vi "Write to Buffer.vi"(7 "clear buffer (False)":bool, 8 "error in (no error)":errorcluster, 9 "timeout (1000 ms)":i32=1000, 10 "waveforms":waveform(dbl)[](array[waveform]), 11 "buffer":refnum<data-value>) -> (0 "error out":errorcluster, 3 "buffer out":refnum<data-value>)   [LabVIEW 2017, in "Waveforms (N Ch).lvclass"]
doc: "Appends waveforms to existing data in a buffer of continuous waveforms. Use this VI to include additional waveforms in the referenced buffer. <B> waveforms</B> must have identical dt and length, and all waveforms must have the same timestamp. If input waveforms are not continuous with waveforms already in the buffer, the <B> buffer</B> will be cleared and replaced with the <B>waveforms</B>."
uses:
  <vilib>/addons/_NISVFA/_Shared subVIs/Data Objects/Waveforms (DBL)/Waveforms (N Ch).lvclass
  C:/Program Files (x86)/National Instruments/LabVIEW 2017/vi.lib/addons/_NISVFA/_Shared subVIs/Data Objects/Data/Data.lvclass
  <vilib>/addons/_NISVFA/_Shared subVIs/Data Objects/Data/Data.lvclass/Data.ctl
  <vilib>/addons/_NISVFA/_Shared subVIs/Data Objects/Waveforms (DBL)/Waveforms (N Ch).lvclass/Waveforms (N Ch).ctl
  <vilib>/addons/_NISVFA/_Shared subVIs/Data Objects/Waveforms (DBL)/Read Mode for Deleting Stale Data.vi
  <vilib>/addons/_NISVFA/_Shared subVIs/Data Objects/Data/Read Channel Length.vi
  <vilib>/addons/_NISVFA/_Shared subVIs/Data Objects/Waveforms (DBL)/Read Maximum Channel Duration.vi
  <vilib>/addons/_NISVFA/_Shared subVIs/Data Objects/Data/Read Maximum Channel Length.vi
  <vilib>/addons/_NISVFA/_Shared subVIs/Data Objects/Data/Read Channel Count.vi
  <vilib>/addons/_NISVFA/_Shared subVIs/Data Objects/subVIs/Get Oldest of ReaderTimestamps.vi
  <vilib>/addons/_NISVFA/_Shared subVIs/Common/SV Get Data Subset.vi
  <vilib>/addons/_NISVFA/_Shared subVIs/Common/svc_Get Waveform Subset (Index).vi
  <vilib>/addons/_NISVFA/_Shared subVIs/Common/sv_Convert Timestamp to Relative Index.vi
  <vilib>/addons/_NISVFA/_Shared subVIs/Common/sv_Get NI Property Name String.vi
  <vilib>/addons/_NISVFA/_Shared subVIs/Common/svc_Check for Waveform Parameter Continuity (no state).vi
  <vilib>/addons/_NISVFA/_Shared subVIs/Data Objects/subVIs/Get Channel Count.vi
  <vilib>/addons/_NISVFA/_Shared subVIs/Common/svc_Get Array Subset (Index).vi
  <vilib>/addons/_NISVFA/_Shared subVIs/Common/svc_Get SV Channel Info.vi
  <vilib>/addons/_NISVFA/_Shared subVIs/Common/svc_Coerce Index and Length.vi
  <vilib>/addons/_NISVFA/_Shared subVIs/Common/svc_Engineering Units to Unit Label.vi
  <vilib>/addons/_NISVFA/_Shared subVIs/Common/svc_Unit Label to Engineering Units.vi
  <vilib>/addons/_NISVFA/_Shared subVIs/Data Objects/subVIs/Get Maximum Data Length.vi
  <vilib>/addons/_NISVFA/_Shared subVIs/Data Objects/subVIs/Get Maximum Data Duration.vi
  <vilib>/ErrorRing/Error Ring.xnode
  <vilib>/addons/_NISVFA/_Shared subVIs/Data Objects/Data/Data.lvclass
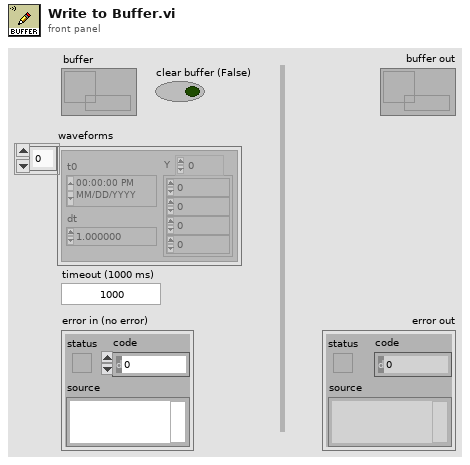
[diagram p1: front panel]
types:
  T1 = typedef "svc_Delete Data Options (enum).ctl" = enum16{"Write", "Read", "Release"}
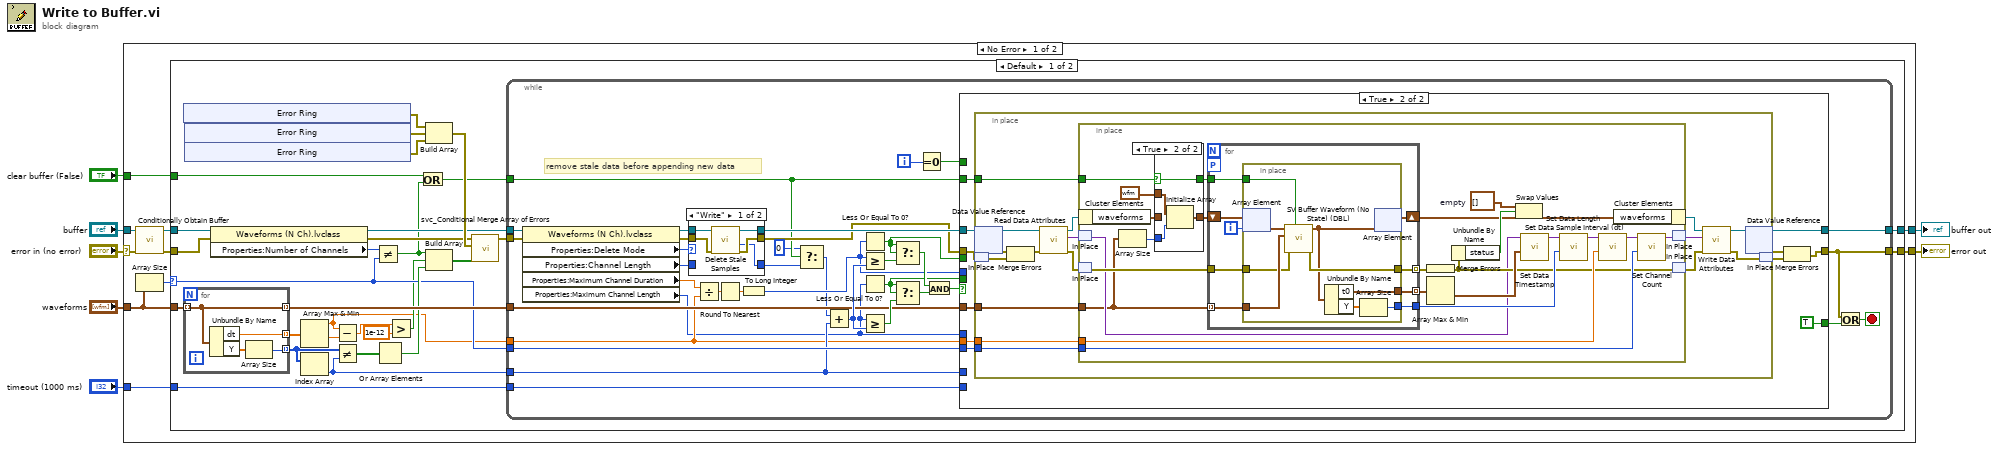
[diagram p0: block diagram]
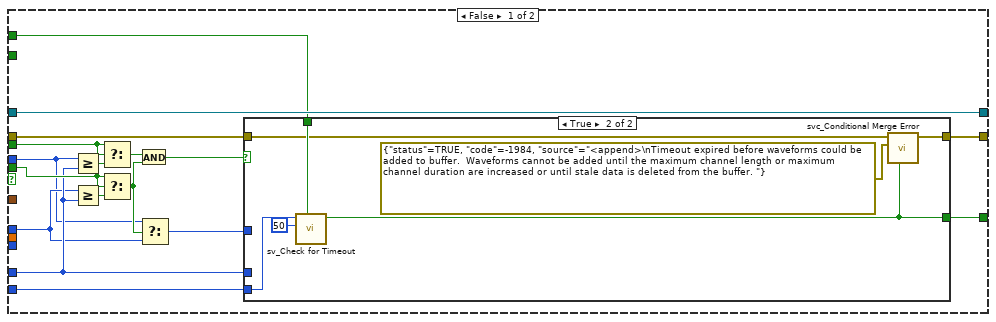
[diagram p2: hidden frame]
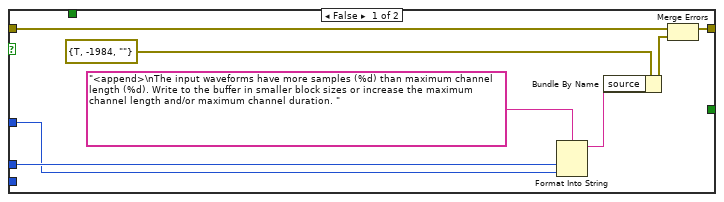
[diagram p3: hidden frame]
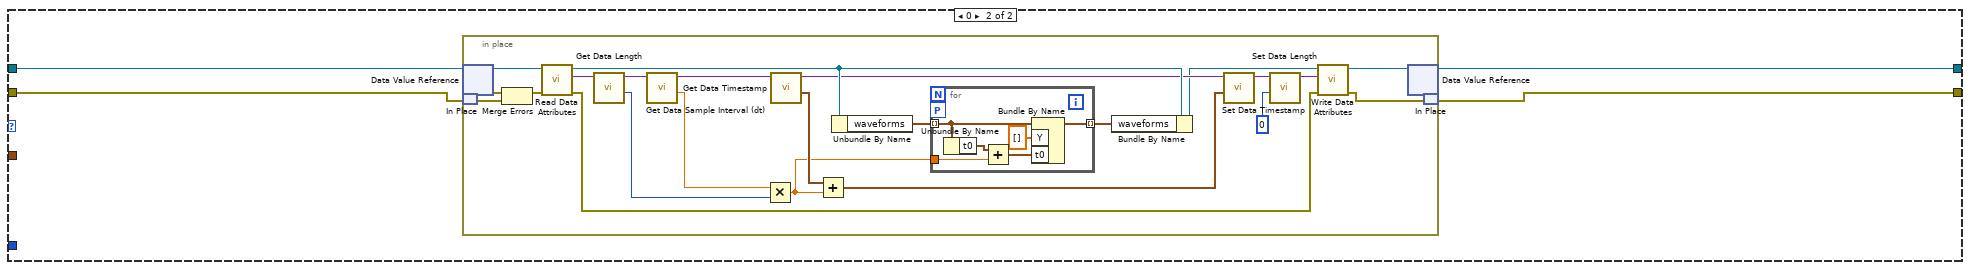
[diagram p6: hidden frame]
diagram:
  n1 = case shown="No Error" "error in (no error)" {
    selector: "error in (no error)" -> [w13 w239]
    tunnel: [w16 w239] -> w6
    tunnel: [w17 w240] -> w2
    tunnel: "buffer" -> [w15 w240]
    tunnel: "waveforms" -> [w11 _]
    tunnel: "clear buffer (False)" -> [w12 _]
    tunnel: "timeout (1000 ms)" -> [w8 _]
    frame No Error {
      n2 = call <vilib>:"Conditionally Obtain Buffer.vi"("error in (no error)"=w13, "buffer"=w15) -> ("error out"=w9:errorcluster, "buffer"=w14:refnum<data-value>)  [unwired: 8 in]
      n3 = Array Size(array=w11) -> (size(s)=w10:i32)
      n4 = case shown="Default" w10 {
        selector: w10 -> [w23 _]
        tunnel: w12 -> [w35 _]
        tunnel: [w46 w208] -> w17
        tunnel: [w47 w206] -> w16
        tunnel: w14 -> [w33 w209]
        tunnel: w11 -> [w45 _]
        tunnel: w9 -> [w32 w207]
        tunnel: w8 -> [w24 _]
        frame Default {
          n5 = xnode "Error Ring"() -> ("error out"=w25:errorcluster)
          n6 = for {
            tunnel: w45 -> [w201] mode=indexing
            tunnel: [w201] -> w44 mode=indexing
            tunnel: [w200] -> w41 mode=indexing
            tunnel: [w199] -> w40 mode=indexing
            n7 = Unbundle By Name(w201) -> ("dt"=w200:dbl, "Y"=w202:dbl[])
            n8 = Array Size(array=w202) -> (size(s)=w199:i32)
          }
          n9 = xnode "Error Ring"() -> ("error out"=w39:errorcluster)
          n10 = xnode "Error Ring"() -> ("error out"=w38:errorcluster)
          n11 = property class="Waveforms (N Ch).lvclass"(reference=w33, error in=w32) -> (reference out=w31:refnum<data-value>, error out=w29:errorcluster, "Properties:Number of Channels"=w30:i32)
          n12 = Array Max & Min(array=w41) -> (max value=w18:dbl, min value=w22:dbl)  [unwired: 2 out]
          n13 = Index Array(array=w40) -> (element=w27:i32)  [unwired: 1 in]
          n14 = Subtract(x=w18, y=w22) -> (x-y=w21:dbl)
          n15 = Not Equal?(x=w40, y=w27) -> (x != y?=w42:bool[])
          n16 = Not Equal?(x=w30, y=w23) -> (x != y?=w26:bool)
          n17 = Or Array Elements(Boolean array=w42) -> (logical OR=w43:bool)
          n18 = Greater?(x=w21, y=1e-12) -> (0:w20:bool)
          n19 = Or(x=w35, y=w26) -> (x .or. y?=w34:bool)
          n20 = Build Array(w25, w39, w38) -> (w37:errorcluster[])
          n21 = Build Array(w26, w20, w43) -> (w36:bool[])
          n22 = call <vilib>:"svc_Conditional Merge Array of Errors.vi"("condition met"=w36, "possible errors and warnings"=w37, "error in"=w29) -> ("error out"=w28:errorcluster)  [unwired: 8 in]
          n23 = while {
            tunnel: [w60] -> w47
            tunnel: [w83] -> w46
            tunnel: w44 -> [w65]
            tunnel: w23 -> [w79]
            tunnel: w18 -> [w54]
            tunnel: w34 -> [w51]
            tunnel: w31 -> [w78]
            tunnel: w28 -> [w77]
            tunnel: w24 -> [w61]
            tunnel: w27 -> [w67]
            i -> [w63]
            stop <- w58 stop-if-true
            # "remove stale data before appending new data"
            n24 = property class="Waveforms (N Ch).lvclass"(reference=w78, error in=w77) -> (reference out=w81:refnum<data-value>, error out=w82:errorcluster, "Properties:Delete Mode"=w80:T1, "Properties:Channel Length"=w52:i32, "Properties:Maximum Channel Duration"=w56:dbl, "Properties:Maximum Channel Length"=w53:i32)
            n25 = case shown="\"Write\"" w80 {
              tunnel: [w195 w198] -> w76
              tunnel: [w194 w197] -> w57
              tunnel: w82 -> [w193 w197]
              tunnel: w81 -> [w192 w198]
              tunnel: w52 -> [_ w196]
              tunnel: [w191 w196] -> w48
              frame "Write" {
                n26 = call <vilib>:"Delete Stale Samples.vi"("error in (no error)"=w193, "buffer"=w192) -> ("error out"=w194:errorcluster, "new channel length"=w191:i32, "buffer"=w195:refnum<data-value>)  [unwired: 6 in, 1 out]
              }
              frame Default {
              }
            }
            n27 = Divide(x=w56, y=w54) -> (x/y=w75:dbl)
            n28 = Round To Nearest(number=w75) -> (nearest integer value=w74:dbl)
            n29 = To Long Integer(number=w74) -> (32bit integer=w55:i32)
            n30 = Select(t=0, s=w51, f=w48) -> (s? t:f=w49:i32)
            n31 = Add(x=w49, y=w67) -> (x+y=w71:i32)
            n32 = Less Or Equal To 0?(x=w55) -> (x <= 0?=w64:bool)
            n33 = Greater Or Equal?(x=w55, y=w71) -> (x >= y?=w73:bool)
            n34 = Less Or Equal To 0?(x=w53) -> (x <= 0?=w66:bool)
            n35 = Greater Or Equal?(x=w53, y=w71) -> (x >= y?=w72:bool)
            n36 = Select(t=w64, s=w64, f=w73) -> (s? t:f=w70:bool)
            n37 = Select(t=w66, s=w66, f=w72) -> (s? t:f=w69:bool)
            n38 = Equal To 0?(x=w63) -> (x = 0?=w62:bool)
            n39 = And(x=w70, y=w69) -> (x .and. y?=w68:bool)
            n40 = case shown="True" w68 {
              tunnel: [w94 w124] -> w60
              tunnel: [w100 w123] -> w83
              tunnel: w65 -> [_ w122]
              tunnel: w79 -> [_ w121]
              tunnel: w54 -> [_ w120]
              tunnel: w51 -> [_ w119]
              tunnel: w76 -> [w100 w118]
              tunnel: w67 -> [w87 _]
              tunnel: w64 -> [w96 _]
              tunnel: w66 -> [w97 _]
              tunnel: w55 -> [w85 _]
              tunnel: w57 -> [w93 w117]
              tunnel: w53 -> [w86 _]
              tunnel: w62 -> [w92 _]
              tunnel: w61 -> [w91 _]
              tunnel: [w90 TRUE ("timeout")] -> w59
              frame False {
                n41 = Greater Or Equal?(x=w85, y=w87) -> (x >= y?=w98:bool)
                n42 = Greater Or Equal?(x=w86, y=w87) -> (x >= y?=w99:bool)
                n43 = Select(t=w96, s=w96, f=w98) -> (s? t:f=w95:bool)
                n44 = Select(t=w97, s=w97, f=w99) -> (s? t:f=w88:bool)
                n45 = And(x=w95, y=w88) -> (x .and. y?=w89:bool)
                n46 = Select(t=w85, s=w88, f=w86) -> (s? t:f=w84:i32)
                n47 = case shown="True" w89 {
                  tunnel: [w107 w111] -> w94
                  tunnel: w93 -> [w108 w112]
                  tunnel: w92 -> [_ w115]
                  tunnel: w91 -> [_ w114]
                  tunnel: [_ w109] -> w90
                  tunnel: w87 -> [w102 _]
                  tunnel: w84 -> [w101 _]
                  frame False {
                    n48 = Format Into String(format string="<append>\nThe input waveforms have more samples (%d) than maximum channel length (%d). Write to the buffer in smaller block sizes or increase the maximum channel length and/or maximum channel duration. ", w102, w101) -> (resulting string=w104:string)  [unwired: 2 in, 1 out]
                    n49 = Bundle By Name(cluster=errorcluster {"status"=TRUE, "code"=-1984, "source"=""} ("error constant"), "source"=w104) -> (w105:errorcluster)
                    n50 = Merge Errors(w108, w105) -> (w107:errorcluster)
                  }
                  frame True {
                    n51 = call <vilib>:"sv_Check for Timeout.vi"("reset"=w115, "polling delay [ms]"=50, "timeout [ms]"=w114) -> ("timeout"=w109:bool)  [unwired: 7 in, 1 out]
                    n52 = call <vilib>:"svc_Conditional Merge Error.vi"("merge"=w109, "new error"=errorcluster {"status"=TRUE, "code"=-1984, "source"="<append>\nTimeout expired before waveforms could be added to buffer.  Waveforms cannot be added until the maximum channel length or maximum channel duration are increased or until stale data is deleted from the buffer. "} ("error constant"), "error in (no error)"=w112) -> ("error out"=w111:errorcluster)  [unwired: 8 in]
                  }
                }
              }
              frame True {
                n53 = in-place {
                  in-place-border: w122 -> [w142]
                  in-place-border: w121 -> [w135]
                  in-place-border: w120 -> [w134]
                  in-place-border: w119 -> [w133]
                  n54 = in-place-dvr #1(w118) -> (w141:refnum<class "Waveforms (N Ch).lvclass">, w140:errorcluster)
                  n55 = in-place-match #2(w117) -> (w139:errorcluster)
                  n56 = Merge Errors(w140, w139) -> (w138:errorcluster)
                  n57 = call <vilib>:"Read Data Attributes.vi"("error in (no error)"=w138, "Data in"=w141) -> ("error out"=w130:errorcluster, "data attributes"=w129:variant, "Data out"=w132:refnum<class "Waveforms (N Ch).lvclass">)  [unwired: 7 in]
                  n58 = in-place {
                    in-place-border: w142 -> [w144]
                    in-place-border: w135 -> [w163]
                    in-place-border: w134 -> [w161]
                    in-place-border: w133 -> [w149]
                    w153 = waveform(dbl)[] []  # empty
                    n59 = in-place-cluster #3(w132) -> ("waveforms"=w145:waveform(dbl)[])
                    n60 = in-place-match #4(w129) -> (w150:variant)
                    n61 = in-place-match #5(w130) -> (w157:errorcluster)
                    n62 = Array Size(array=w144) -> (size(s)=w143:i32)
                    n63 = case shown="True" w149 {
                      selector: w149 -> [w168 w172]
                      tunnel: [w168 w172] -> w148
                      tunnel: [w167 w170] -> w147
                      tunnel: waveform(dbl) {"t0"=timestamp(0 s since 1904-01-01), "dt"=1.0, "Y"=[]} ("buffer out") -> [_ w171]
                      tunnel: w145 -> [w167 _]
                      tunnel: w143 -> [_ w169]
                      frame False {
                      }
                      frame True {
                        n64 = Initialize Array(w171, w169) -> (w170:waveform(dbl)[])
                      }
                    }
                    n65 = for {
                      tunnel: w144 -> [w181] mode=indexing
                      tunnel: w148 -> [w180]
                      tunnel: [w179] -> w164 mode=indexing
                      tunnel: [w178] -> w162 mode=indexing
                      tunnel: w157 -> [w177]
                      tunnel: [w176] -> w166
                      shift-right: [w173] -> w152
                      shift-left: w147 -> [w174]
                      workers-P: _ -> [_]
                      i -> [w175]
                      n66 = in-place {
                        in-place-border: w181 -> [w190]
                        in-place-border: w180 -> [w189]
                        in-place-border: [w188] -> w179
                        in-place-border: [w186] -> w178
                        in-place-border: w177 -> [w185]
                        in-place-border: [w184] -> w176
                        n67 = in-place-array #6(w174, w175) -> (w183:waveform(dbl))
                        n68 = call <vilib>:"SV Buffer Waveform (No State) (DBL).vi"("clear buffer (False)"=w189, "error in (no error)"=w185, "waveform"=w190, "buffer in"=w183) -> ("error out"=w186:errorcluster, "buffer out"=w182:waveform(dbl))  [unwired: 6 in]
                        n69 = Unbundle By Name(w182) -> ("t0"=w188:timestamp, "Y"=w187:dbl[])
                        n70 = Array Size(array=w187) -> (size(s)=w184:i32)
                        n71 = in-place-array #6(w182) -> (w173:waveform(dbl)[])  [unwired: 1 out]
                      }
                    }
                    n72 = Merge Errors(w162) -> (w155:errorcluster)
                    n73 = Array Max & Min(array=w164) -> (min value=w165:timestamp)  [unwired: 3 out]
                    n74 = Unbundle By Name(w155) -> ("status"=w154:bool)
                    n75 = Swap Values(12:w153, 13:w154, 14:w152) -> (3:w151:waveform(dbl)[])  [unwired: 1 out]
                    n76 = call <vilib>:"Set Data Timestamp.vi"("timestamp"=w165, "variant in"=w150) -> ("variant out"=w160:variant)  [unwired: 9 in]
                    n77 = call <vilib>:"Set Data Length.vi"("number of samples"=w166, "variant in"=w160) -> ("variant out"=w159:variant)  [unwired: 9 in]
                    n78 = call <vilib>:"Set Data Sample Interval (dt).vi"("dt [s]"=w161, "variant in"=w159) -> ("variant out"=w158:variant)  [unwired: 9 in]
                    n79 = in-place-cluster #3("waveforms"=w151) -> (w131:refnum<class "Waveforms (N Ch).lvclass">)
                    n80 = call <vilib>:"Set Channel Count.vi"("number of channels"=w163, "variant in"=w158) -> ("variant out"=w156:variant)  [unwired: 9 in]
                    n81 = in-place-match #4(w156) -> (w128:variant)
                    n82 = in-place-match #5(w155) -> (w127:errorcluster)
                  }
                  n83 = call <vilib>:"Write Data Attributes.vi"("error in (no error)"=w127, "data attributes"=w128, "Data in"=w131) -> ("error out"=w136:errorcluster, "Data out"=w137:refnum<class "Waveforms (N Ch).lvclass">)  [unwired: 7 in]
                  n84 = in-place-dvr #1(w137) -> (w123:refnum<data-value>, w126:errorcluster)
                  n85 = in-place-match #2(w136) -> (w125:errorcluster)
                }
                n86 = Merge Errors(w126, w125) -> (w124:errorcluster)
              }
            }
            n87 = Or(x=w60, y=w59) -> (x .or. y?=w58:bool)
          }
        }
        frame 0 {
          n88 = in-place {
            n89 = in-place-dvr #7(w209) -> (w232:refnum<class "Waveforms (N Ch).lvclass">, w231:errorcluster)
            n90 = in-place-match #8(w207) -> (w230:errorcluster)
            n91 = Merge Errors(w231, w230) -> (w229:errorcluster)
            n92 = call <vilib>:"Read Data Attributes.vi"("error in (no error)"=w229, "Data in"=w232) -> ("error out"=w227:errorcluster, "data attributes"=w223:variant, "Data out"=w228:refnum<class "Waveforms (N Ch).lvclass">)  [unwired: 7 in]
            n93 = call <vilib>:"Get Data Length.vi"("variant in"=w223) -> ("number of samples"=w221:i32, "variant out"=w224:variant)  [unwired: 9 in]
            n94 = call <vilib>:"Get Data Sample Interval (dt).vi"("variant in"=w224) -> ("dt [s]"=w220:dbl, "variant out"=w222:variant)  [unwired: 9 in]
            n95 = Multiply(x=w220, y=w221) -> (x*y=w217:dbl)
            n96 = call <vilib>:"Get Data Timestamp.vi"("variant in"=w222) -> ("timestamp"=w219:timestamp, "variant out"=w226:variant)  [unwired: 9 in]
            n97 = Add(x=w219, y=w217) -> (x+y=w218:timestamp)
            n98 = Unbundle By Name(w228) -> ("waveforms"=w212:waveform(dbl)[])
            n99 = for {
              tunnel: w212 -> [w236] mode=indexing
              tunnel: [w237] -> w211 mode=indexing
              tunnel: w217 -> [w234]
              workers-P: _ -> [_]
              n100 = Unbundle By Name(w236) -> ("t0"=w235:timestamp)
              n101 = Add(x=w235, y=w234) -> (x+y=w233:timestamp)
              n102 = Bundle By Name(cluster=w236, "Y"=dbl[] [], "t0"=w233) -> (w237:waveform(dbl))
            }
            n103 = Bundle By Name(cluster=w228, "waveforms"=w211) -> (w216:refnum<class "Waveforms (N Ch).lvclass">)
            n104 = call <vilib>:"Set Data Timestamp.vi"("timestamp"=w218, "variant in"=w226) -> ("variant out"=w215:variant)  [unwired: 9 in]
            n105 = call <vilib>:"Set Data Length.vi"("number of samples"=0, "variant in"=w215) -> ("variant out"=w214:variant)  [unwired: 9 in]
            n106 = call <vilib>:"Write Data Attributes.vi"("error in (no error)"=w227, "data attributes"=w214, "Data in"=w216) -> ("error out"=w210:errorcluster, "Data out"=w225:refnum<class "Waveforms (N Ch).lvclass">)  [unwired: 7 in]
            n107 = in-place-dvr #7(w225) -> (w208:refnum<data-value>)  [unwired: 1 out]
            n108 = in-place-match #8(w210) -> (w206:errorcluster)
          }
        }
      }
    }
    frame Error {
    }
  }
  "error out" <- w6
  "buffer out" <- w2
